vi "Calculate Shortest Move.vi"(9 "Target Filter":i32, 10 "Curr Filter":i32, 11 "Wheel info":T1) -> (0 "notches":i32, 1 "Msg":string, 2 "direction":bool, 3 "Moves":i32[](array[numeric]))   [LabVIEW 2022 SP3, in "FW Arduino Control.lvclass"]
uses:
  FW Arduino Control.lvclass
  Filter Wheel Object/Filter Wheel Details.ctl
  <vilib>/Utility/error.llb/Trim Whitespace One-Sided.vi
  Filter Wheel Object/Filter Wheel.lvclass
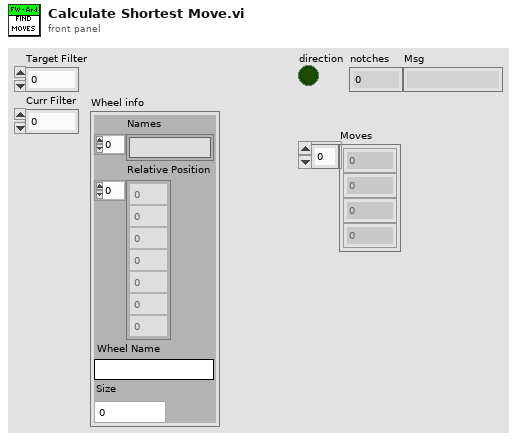
[diagram p1: front panel]
types:
  T1 = typedef "Filter Wheel.lvclass/Filter Wheel Details.ctl" = cluster{"Names":string[], "Relative Position":i32[], "Wheel Name":string, "Size":i32}
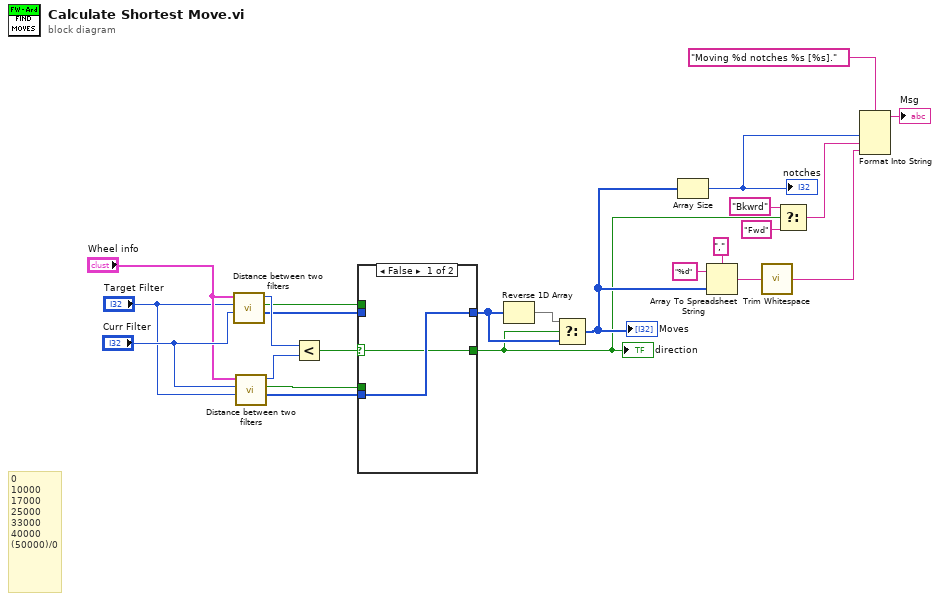
[diagram p0: block diagram]
diagram:
  # "0\n10000\n17000\n25000\n33000\n40000\n(50000)/0"
  n1 = call "Distance between two filters.vi"("End Filter"="Curr Filter", "Start Filter"="Target Filter", "Wheel info"="Wheel info") -> ("Moves"=w17:i32[], "wrap"=w18:bool, "Distance"=w24:i32)  [unwired: 6 in]
  n2 = call "Distance between two filters.vi"("End Filter"="Target Filter", "Start Filter"="Curr Filter", "Wheel info"="Wheel info") -> ("Moves"=w15:i32[], "wrap"=w16:bool, "Distance"=w23:i32)  [unwired: 6 in]
  n3 = Less?(x=w24, y=w23) -> (x < y?=w19:bool)
  n4 = case shown="False" w19 {
    selector: w19 -> [w25 w27]
    tunnel: w18 -> [_ _]
    tunnel: w17 -> [_ w28]
    tunnel: [w26 w28] -> w14
    tunnel: [w25 w27] -> w4
    tunnel: w16 -> [_ _]
    tunnel: w15 -> [w26 _]
    frame False {
    }
    frame True {
    }
  }
  "direction" <- w4
  n5 = Reverse 1D Array(array=w14) -> (reversed array=w13:i32[])
  n6 = Select(t=w13, s=w4, f=w14) -> (s? t:f=w5:i32[])
  "Moves" <- w5
  n7 = Array Size(array=w5) -> (size(s)=w11:i32)
  "notches" <- w11
  n8 = Array To Spreadsheet String(delimiter (Tab)=",", array=w5, 3:"%d" ("format string")) -> (spreadsheet string=w8:string)
  n9 = call <vilib>:"Trim Whitespace.vi"("string"=w8) -> ("trimmed string"=w7:string)  [unwired: 1 in]
  n10 = Select(t="Bkwrd", s=w4, f="Fwd") -> (s? t:f=w6:string)
  n11 = Format Into String(format string="Moving %d notches %s [%s].", w11, w6, w7) -> (resulting string=→"Msg":string)  [unwired: 2 in, 1 out]
